vi "Pack LLP Packet to DRAM Word.vi"(0 "timestamped llp packet":T2, 1 "reset":bool, 2 "flush":bool, 9 "input valid":bool, 11 "count packet size":bool, 12 "ready for output":bool=TRUE) -> (3 "flush complete":bool, 4 "dram word":T1, 6 "valid packet words":u64, 8 "in reset":bool, 10 "output valid":bool, 14 "ready for input":bool, 15 "packet word size":u16)   [LabVIEW 2020, in "GettingStarted_Acq_Tap_148X_FPGA.lvlib"]
uses:
  GettingStarted_Acq_Tap_148X_FPGA.lvlib
  <instrlib>/FlexRIO/CSI-2/v2/FPGA/Types/Timestamped LLP Packet.ctl
  <instrlib>/FlexRIO/CSI-2/v2/FPGA/Types/FPGA LLP Packet Timestamp.ctl
  <instrlib>/FlexRIO/CSI-2/v2/FPGA/Types/Timestamp ID.ctl
  <instrlib>/FlexRIO/CSI-2/v2/FPGA/Types/LLP Packet.ctl
  <instrlib>/FlexRIO/CSI-2/v2/FPGA/Types/LLP Packet Header.ctl
  <instrlib>/FlexRIO/CSI-2/v2/FPGA/Types/LLP Packet Payload.ctl
  <instrlib>/FlexRIO/CSI-2/v2/FPGA/Types/LLP Packet Footer.ctl
  <instrlib>/_niInstr/Memory/v1/FPGA/Memory/Public/U256.ctl
  <instrlib>/FlexRIO/CSI-2/v2/FPGA/Types/Tagged LLP Packet.ctl
  <instrlib>/FlexRIO/CSI-2/v2/FPGA/Types/FPGA LLP Packet Tag.ctl
  <instrlib>/FlexRIO/CSI-2/v2/FPGA/Types/FPGA LLP Packet Size.ctl
  c350671c-88b9-4867-b70d-17d94c71bae3.vi
  6f151b37-587e-4501-b3b8-9b94e7855677.vi
  <instrlib>/_niInstr/Basic Elements/v1/FPGA/Private/Count Up U64.vi
  <instrlib>/_niInstr/Data Formatting/v1/FPGA/Private/Convert/U8 array to Boolean Array.vi
  32b7dccb-5314-4a3c-8b3a-36354efc8b88.vi
  <instrlib>/_niInstr/Data Formatting/v1/FPGA/Private/Pack/Pack Impl.vi
  2704c8c1-3016-4f8b-8a1b-ab3ce532af0c.vi
  <instrlib>/_niInstr/Data Formatting/v1/FPGA/niInstr Data Formatting v1 FPGA.lvlib
  <instrlib>/_niInstr/Memory/v1/FPGA/Memory/niInstr Memory v1 FPGA.lvclass
  <instrlib>/FlexRIO/CSI-2/v2/FPGA/NI CSI-2 API FPGA v2.lvlib
  <instrlib>/_niInstr/Basic Elements/v1/FPGA/niInstr Basic Elements v1 FPGA.lvlib
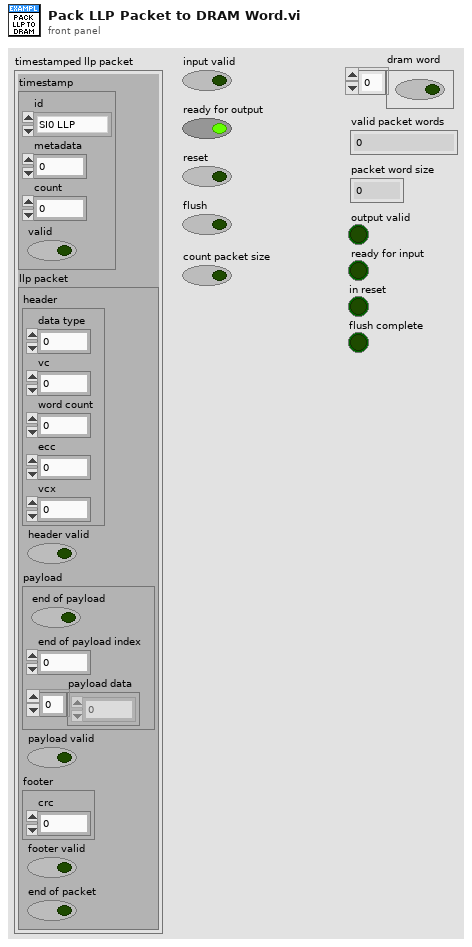
[diagram p1: front panel]
types:
  T1 = typedef "niInstr Memory v1 FPGA.lvclass/U256.ctl" = bool[]
  T2 = typedef "NI CSI-2 API FPGA v2.lvlib/Timestamped LLP Packet.ctl" = cluster{"timestamp":T3, "llp packet":T5}
  T3 = typedef "NI CSI-2 API FPGA v2.lvlib/FPGA LLP Packet Timestamp.ctl" = cluster{"valid":bool, "count":fxp<+,50,50>, "id":T4, "metadata":u8}
  T4 = typedef "NI CSI-2 API FPGA v2.lvlib/Timestamp ID.ctl" = enum8{"SI0 LLP", "SI1 LLP", "SI2 LLP", "SI3 LLP", "SI4 LLP", "SI5 LLP", "SI6 LLP", "SI7 LLP", "SO0 LLP", "SO1 LLP", "SO2 LLP", "SO3 LLP", "SO4 LLP", "SO5 LLP", "SO6 LLP", "SO7 LLP", "Ser0 GPIO Bank", "Ser1 GPIO Bank", "Ser2 GPIO Bank", "Ser3 GPIO Bank", "Ser4 GPIO Bank", "Ser5 GPIO Bank", "Ser6 GPIO Bank", "Ser7 GPIO Bank", "Des0 GPIO Bank", "Des1 GPIO Bank", "Des2 GPIO Bank", "Des3 GPIO Bank", "Des4 GPIO Bank", "Des5 GPIO Bank", "Des6 GPIO Bank", "Des7 GPIO Bank", "User0", "User1", "User2", "User3", "User4", "User5", "User6", "User7", "User8", "User9", "User10", "User11", "User12", "User13", "User14", "User15", "User16", "User17", "User18", "User19", "User20", "User21", "User22", "User23", "User24", "User25", "User26", "User27", "User28", "User29", "User30", "User31"}
  T5 = typedef "NI CSI-2 API FPGA v2.lvlib/LLP Packet.ctl" = cluster{"header":T6, "header valid":bool, "payload":T7, "payload valid":bool, "footer":T8, "footer valid":bool, "end of packet":bool}
  T6 = typedef "NI CSI-2 API FPGA v2.lvlib/LLP Packet Header.ctl" = cluster{"word count":u16, "ecc":fxp<+,6,6>, "vcx":fxp<+,2,2>, "data type":fxp<+,6,6>, "vc":fxp<+,2,2>}
  T7 = typedef "NI CSI-2 API FPGA v2.lvlib/LLP Packet Payload.ctl" = cluster{"end of payload":bool, "end of payload index":fxp<+,3,3>, "payload data":u8[]}
  T8 = typedef "NI CSI-2 API FPGA v2.lvlib/LLP Packet Footer.ctl" = cluster{"crc":u16}
  T9 = typedef "NI CSI-2 API FPGA v2.lvlib/Tagged LLP Packet.ctl" = cluster{"tag":T10, "llp packet":T5}
  T10 = typedef "NI CSI-2 API FPGA v2.lvlib/FPGA LLP Packet Tag.ctl" = cluster{"timestamp":T3, "size":T11}
  T11 = typedef "NI CSI-2 API FPGA v2.lvlib/FPGA LLP Packet Size.ctl" = cluster{"bytes":fxp<+,17,17>, "valid":bool}
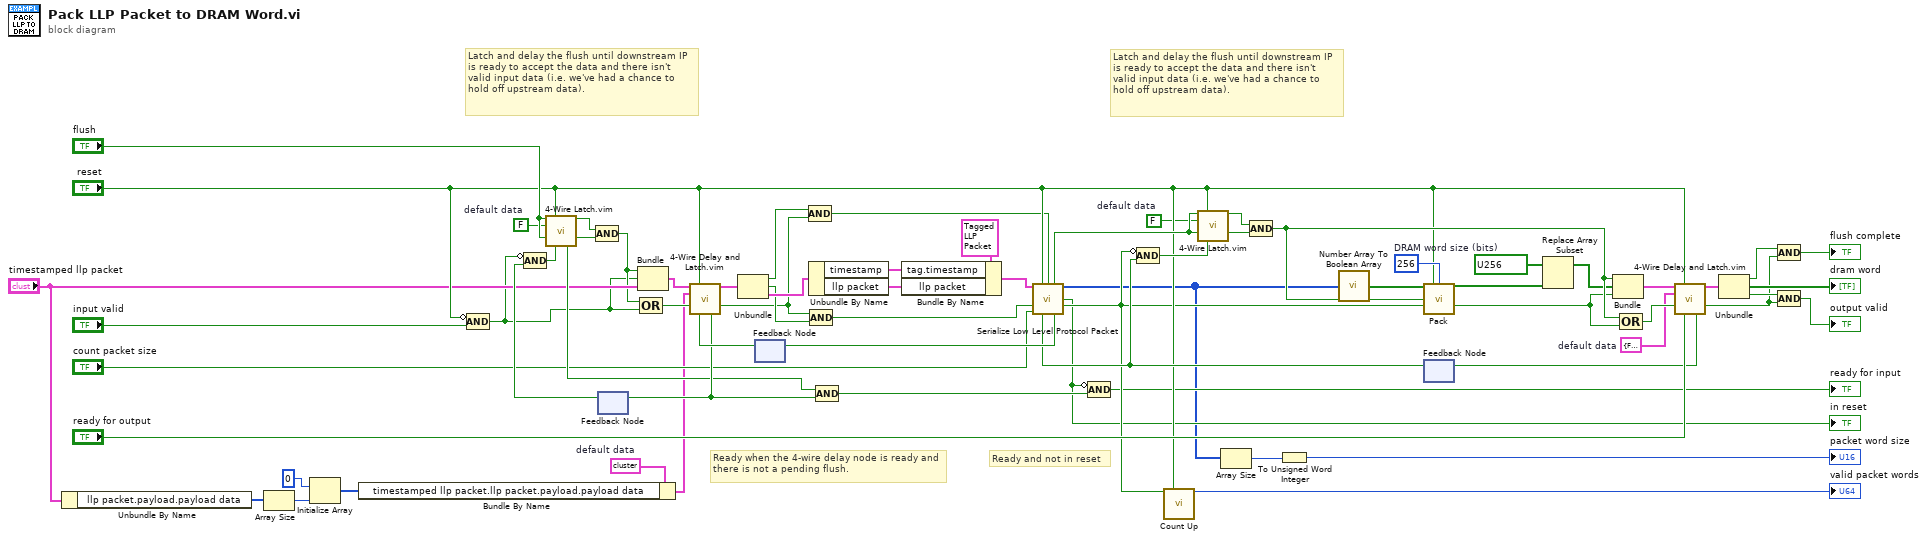
[diagram p0: block diagram]
diagram:
  w7 = cluster{bool, bool, "timestamped llp packet":T2} {FALSE, FALSE, "timestamped llp packet"={"timestamp"={"valid"=FALSE, "count"=0.0, "id"=enum."SI0 LLP", "metadata"=0}, "llp packet"={"header"={"word count"=0, "ecc"=0.0, "vcx"=0.0, "data type"=0.0, "vc"=0.0}, "header valid"=FALSE, "payload"={"end of payload"=FALSE, "end of payload index"=0.0, "payload data"=[]}, "payload valid"=FALSE, "footer"={"crc"=0}, "footer valid"=FALSE, "end of packet"=FALSE}}}  # default data
  w10 = cluster{bool, "data":T1, "output valid":bool} {FALSE, "data"=[FALSE, FALSE, FALSE, FALSE, FALSE, FALSE, FALSE, FALSE, FALSE, FALSE, FALSE, FALSE, FALSE, FALSE, FALSE, FALSE, FALSE, FALSE, FALSE, FALSE, FALSE, FALSE, FALSE, FALSE, FALSE, FALSE, FALSE, FALSE, FALSE, FALSE, FALSE, FALSE, FALSE, FALSE, FALSE, FALSE, FALSE, FALSE, FALSE, FALSE, FALSE, FALSE, FALSE, FALSE, FALSE, FALSE, FALSE, FALSE, FALSE, FALSE, FALSE, FALSE, FALSE, FALSE, FALSE, FALSE, FALSE, FALSE, FALSE, FALSE, FALSE, FALSE, FALSE, FALSE, FALSE, FALSE, FALSE, FALSE, FALSE, FALSE, FALSE, FALSE, FALSE, FALSE, FALSE, FALSE, FALSE, FALSE, FALSE, FALSE, FALSE, FALSE, FALSE, FALSE, FALSE, FALSE, FALSE, FALSE, FALSE, FALSE, FALSE, FALSE, FALSE, FALSE, FALSE, FALSE, FALSE, FALSE, FALSE, FALSE, FALSE, FALSE, FALSE, FALSE, FALSE, FALSE, FALSE, FALSE, FALSE, FALSE, FALSE, FALSE, FALSE, FALSE, FALSE, FALSE, FALSE, FALSE, FALSE, FALSE, FALSE, FALSE, FALSE, FALSE, FALSE, FALSE, FALSE, FALSE, FALSE, FALSE, FALSE, FALSE, FALSE, FALSE, FALSE, FALSE, FALSE, FALSE, FALSE, FALSE, FALSE, FALSE, FALSE, FALSE, FALSE, FALSE, FALSE, FALSE, FALSE, FALSE, FALSE, FALSE, FALSE, FALSE, FALSE, FALSE, FALSE, FALSE, FALSE, FALSE, FALSE, FALSE, FALSE, FALSE, FALSE, FALSE, FALSE, FALSE, FALSE, FALSE, FALSE, FALSE, FALSE, FALSE, FALSE, FALSE, FALSE, FALSE, FALSE, FALSE, FALSE, FALSE, FALSE, FALSE, FALSE, FALSE, FALSE, FALSE, FALSE, FALSE, FALSE, FALSE, FALSE, FALSE, FALSE, FALSE, FALSE, FALSE, FALSE, FALSE, FALSE, FALSE, FALSE, FALSE, FALSE, FALSE, FALSE, FALSE, FALSE, FALSE, FALSE, FALSE, FALSE, FALSE, FALSE, FALSE, FALSE, FALSE, FALSE, FALSE, FALSE, FALSE, FALSE, FALSE, FALSE, FALSE, FALSE, FALSE, FALSE, FALSE, FALSE, FALSE, FALSE, FALSE, FALSE, FALSE, FALSE, FALSE, FALSE, FALSE, FALSE, FALSE, FALSE, FALSE, FALSE, FALSE, FALSE, FALSE, FALSE, FALSE, FALSE, FALSE, FALSE, FALSE, FALSE, FALSE], "output valid"=FALSE}  # default data
  w17 = FALSE  # default data
  w18 = FALSE  # default data
  w67 = u16 256  # DRAM word size (bits)
  # "Ready and not in reset"
  # "Ready when the 4-wire delay node is ready and there is not a pending flush."
  # "Latch and delay the flush until downstream IP is ready to accept the data and there isn't valid input data (i.e. we've had a chance to hold off upstream data)."
  # "Latch and delay the flush until downstream IP is ready to accept the data and there isn't valid input data (i.e. we've had a chance to hold off upstream data)."
  n1 = Unbundle By Name("timestamped llp packet") -> ("llp packet.payload.payload data"=w14:u8[])
  n2 = Array Size(array=w14) -> (size(s)=w13:i32)
  n3 = Initialize Array(u8 0 ("element"), w13) -> (w11:u8[])
  n4 = Bundle By Name(cluster=w7, "timestamped llp packet.llp packet.payload.payload data"=w11) -> (w15:cluster{bool, bool, "timestamped llp packet":T2})
  n5 = Compound Arithmetic op=AND(invert "reset", "input valid") -> (w8:bool)
  n6 = feedback #1() -> (w57:bool)  [unwired: 1 in]
  n7 = Compound Arithmetic op=AND(invert w8, w57) -> (w58:bool)
  n8 = call "4-Wire Latch.vim"("data in"="flush", "reset"="reset", "default data"=w18, "input valid"="flush", "ready for output"=w58) -> ("data out"=w60:bool, "output valid"=w59:bool, "ready for input"=w35:bool)  [unwired: 8 in]
  n9 = Compound Arithmetic op=AND(w60, w59) -> (w9:bool)
  n10 = Bundle(w9, w8, "timestamped llp packet"="timestamped llp packet") -> (w55:cluster{bool, bool, "timestamped llp packet":T2})  [unwired: 1 in]
  n11 = Compound Arithmetic op=OR(w9, w8) -> (w56:bool)
  n12 = feedback #2() -> (w62:bool)  [unwired: 1 in]
  n13 = call "4-Wire Delay and Latch.vim"("data in"=w55, "reset"="reset", "default data"=w15, "input valid"=w56, "ready for output"=w62) -> ("data out"=w65:cluster{bool, bool, "timestamped llp packet":T2}, "output valid"=w2:bool, "ready for input"=w43:bool)  [unwired: 8 in]
  n14 = feedback-in #1(w43) -> ()
  n15 = Unbundle(w65) -> (w4:bool, w5:bool, "timestamped llp packet"=w6:T2)
  n16 = Compound Arithmetic op=AND(w4, w2) -> (w3:bool)
  n17 = Unbundle By Name(w6) -> ("timestamp"=w33:T3, "llp packet"=w32:T5)
  n18 = Compound Arithmetic op=AND(w2, w5) -> (w1:bool)
  n19 = Compound Arithmetic op=AND(w35, w43) -> (w42:bool)
  n20 = Bundle By Name(cluster=T9 {"tag"={"timestamp"={"valid"=FALSE, "count"=0.0, "id"=enum."SI0 LLP", "metadata"=0}, "size"={"bytes"=0.0, "valid"=FALSE}}, "llp packet"={"header"={"word count"=0, "ecc"=0.0, "vcx"=0.0, "data type"=0.0, "vc"=0.0}, "header valid"=FALSE, "payload"={"end of payload"=FALSE, "end of payload index"=0.0, "payload data"=[0, 0, 0, 0]}, "payload valid"=FALSE, "footer"={"crc"=0}, "footer valid"=FALSE, "end of packet"=FALSE}} ("Metadata LLP Packet"), "tag.timestamp"=w33, "llp packet"=w32) -> (w31:T9)
  n21 = feedback #3() -> (w49:bool)  [unwired: 1 in]
  n22 = call "Serialize Low Level Protocol Packet.vi"("tagged llp packet"=w31, "reset"="reset", "flush"=w3, "input valid"=w1, "count packet size"="count packet size", "ready for output"=w49) -> ("flush complete"=w50:bool, "serialized data"=w21:u8[], "in reset"=w22:bool, "output valid"=w29:bool, "ready for input"=w61:bool)  [unwired: 3 in, 2 out]
  "in reset" <- w22
  n23 = feedback-in #2(w61) -> ()
  n24 = Compound Arithmetic op=AND(invert w22, w42) -> (→"ready for input":bool)
  n25 = Compound Arithmetic op=AND(invert w29, w49) -> (w51:bool)
  n26 = call-poly <instrlib>:"Count Up.vi"("increment"=w29, "reset"="reset") -> ("count out"=→"valid packet words":u64)  [unwired: 13 in]
  n27 = call "4-Wire Latch.vim"("data in"=w50, "reset"="reset", "default data"=w17, "input valid"=w50, "ready for output"=w51) -> ("data out"=w53:bool, "output valid"=w52:bool)  [unwired: 8 in, 1 out]
  n28 = Array Size(array=w21) -> (size(s)=w20:i32)
  n29 = Compound Arithmetic op=AND(w53, w52) -> (w47:bool)
  n30 = To Unsigned Word Integer(number=w20) -> (unsigned 16bit integer=→"packet word size":u16)
  n31 = call-poly <instrlib>:"Number Array To Boolean Array.vi"("data in"=w21) -> ("data out"=w66:bool[])  [unwired: 14 in]
  n32 = call-poly <instrlib>:"Pack.vi"("data in"=w66, "reset"="reset", "number of output data elements"=w67, "flush data"=w47, "input valid"=w29) -> ("data out"=w26:bool[], "output valid"=w39:bool)  [unwired: 7 in, 2 out]
  n33 = Replace Array Subset(array=T1 [FALSE, FALSE, FALSE, FALSE, FALSE, FALSE, FALSE, FALSE, FALSE, FALSE, FALSE, FALSE, FALSE, FALSE, FALSE, FALSE, FALSE, FALSE, FALSE, FALSE, FALSE, FALSE, FALSE, FALSE, FALSE, FALSE, FALSE, FALSE, FALSE, FALSE, FALSE, FALSE, FALSE, FALSE, FALSE, FALSE, FALSE, FALSE, FALSE, FALSE, FALSE, FALSE, FALSE, FALSE, FALSE, FALSE, FALSE, FALSE, FALSE, FALSE, FALSE, FALSE, FALSE, FALSE, FALSE, FALSE, FALSE, FALSE, FALSE, FALSE, FALSE, FALSE, FALSE, FALSE, FALSE, FALSE, FALSE, FALSE, FALSE, FALSE, FALSE, FALSE, FALSE, FALSE, FALSE, FALSE, FALSE, FALSE, FALSE, FALSE, FALSE, FALSE, FALSE, FALSE, FALSE, FALSE, FALSE, FALSE, FALSE, FALSE, FALSE, FALSE, FALSE, FALSE, FALSE, FALSE, FALSE, FALSE, FALSE, FALSE, FALSE, FALSE, FALSE, FALSE, FALSE, FALSE, FALSE, FALSE, FALSE, FALSE, FALSE, FALSE, FALSE, FALSE, FALSE, FALSE, FALSE, FALSE, FALSE, FALSE, FALSE, FALSE, FALSE, FALSE, FALSE, FALSE, FALSE, FALSE, FALSE, FALSE, FALSE, FALSE, FALSE, FALSE, FALSE, FALSE, FALSE, FALSE, FALSE, FALSE, FALSE, FALSE, FALSE, FALSE, FALSE, FALSE, FALSE, FALSE, FALSE, FALSE, FALSE, FALSE, FALSE, FALSE, FALSE, FALSE, FALSE, FALSE, FALSE, FALSE, FALSE, FALSE, FALSE, FALSE, FALSE, FALSE, FALSE, FALSE, FALSE, FALSE, FALSE, FALSE, FALSE, FALSE, FALSE, FALSE, FALSE, FALSE, FALSE, FALSE, FALSE, FALSE, FALSE, FALSE, FALSE, FALSE, FALSE, FALSE, FALSE, FALSE, FALSE, FALSE, FALSE, FALSE, FALSE, FALSE, FALSE, FALSE, FALSE, FALSE, FALSE, FALSE, FALSE, FALSE, FALSE, FALSE, FALSE, FALSE, FALSE, FALSE, FALSE, FALSE, FALSE, FALSE, FALSE, FALSE, FALSE, FALSE, FALSE, FALSE, FALSE, FALSE, FALSE, FALSE, FALSE, FALSE, FALSE, FALSE, FALSE, FALSE, FALSE, FALSE, FALSE, FALSE, FALSE, FALSE, FALSE, FALSE, FALSE, FALSE, FALSE, FALSE, FALSE, FALSE, FALSE, FALSE, FALSE, FALSE, FALSE, FALSE, FALSE, FALSE, FALSE, FALSE, FALSE, FALSE] ("data"), new element=w26) -> (w25:T1)  [unwired: 1 in]
  n34 = Bundle(w47, "data"=w25, "output valid"=w39) -> (w48:cluster{bool, "data":T1, "output valid":bool})  [unwired: 1 in]
  n35 = Compound Arithmetic op=OR(w47, w39) -> (w46:bool)
  n36 = call "4-Wire Delay and Latch.vim"("data in"=w48, "reset"="reset", "default data"=w10, "input valid"=w46, "ready for output"="ready for output") -> ("data out"=w45:cluster{bool, "data":T1, "output valid":bool}, "output valid"=w36:bool, "ready for input"=w63:bool)  [unwired: 8 in]
  n37 = feedback-in #3(w63) -> ()
  n38 = Unbundle(w45) -> (w41:bool, "data"=→"dram word":T1, "output valid"=w38:bool)
  n39 = Compound Arithmetic op=AND(w41, w36) -> (→"flush complete":bool)
  n40 = Compound Arithmetic op=AND(w38, w36) -> (→"output valid":bool)
